vi "Side Convertor.vi"(11 "LV side":T2=1 items=["Left"=1, "Right"=0]) -> (3 "side":T1=141 items=["CblasLeft"=141, "CblasRight"=142])   [LabVIEW 2018, in "NI_AALBLAS.lvlib"]
uses:
  NI_AALBLAS.lvlib
  LV_Side.ctl
  Side.ctl
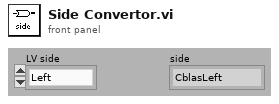
[diagram p1: front panel]
types:
  T1 = typedef "NI_AALBLAS.lvlib/Side.ctl" = i32
  T2 = typedef "NI_AALBLAS.lvlib/LV_Side.ctl" = i32
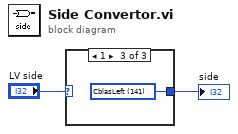
[diagram p0: block diagram]
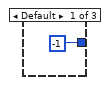
[diagram p2: hidden frame]
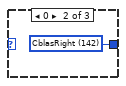
[diagram p3: hidden frame]
diagram:
  n1 = case shown="1" "LV side" {
    tunnel: [-1 w4 w5] -> w2
    frame Default {
    }
    frame 0 {
      w4 = T1 142 items=["CblasLeft"=141, "CblasRight"=142] ("side 2")
    }
    frame 1 {
      w5 = T1 141 items=["CblasLeft"=141, "CblasRight"=142] ("side 2")
    }
  }
  "side" <- w2
